vi "Configure Control AO Split.vi"(0 "VISA resource name":refnum<visa-resource-name>, 1 "Output 0% value of Line Point":dbl min=-1000.0 max=2000.0 step=1.0 format="%.1f", 5 "Unit No. (0)":i32 min=0 max=6, 7 "Module No.(0)":i32 min=0 max=9, 9 "AO No.(1)":i32=1 min=1 max=2, 11 "error in (no error)":errorcluster, 12 "Line Mode(false)":bool, 13 "Output 100% value of Line Point":dbl=100.0 min=-1000.0 max=2000.0 format="%.1f") -> (4 "VISA resource name out":refnum<visa-resource-name>, 6 "AO No.":i32, 8 "Unit No.":i32, 10 "Module No.":i32, 15 "error out":errorcluster)   [LabVIEW 2020, in "Yokogawa GX Series.lvlib"]
doc: "Set AO Split of the PID Module.\n\nCommand: SCtrlSplitAO"
uses:
  <instrlib>/Yokogawa GX Series/Yokogawa GX Series.lvlib
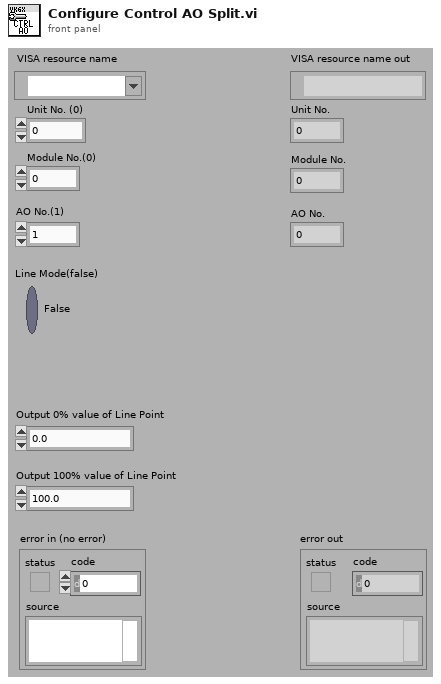
[diagram p1: front panel]
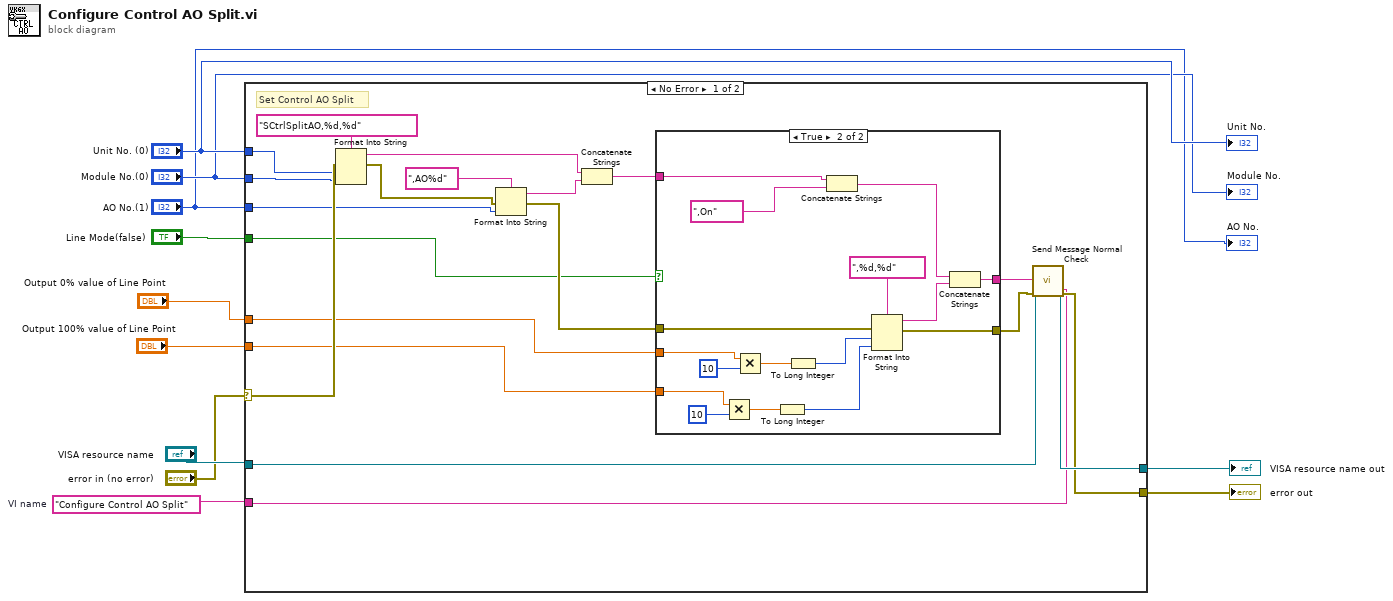
[diagram p0: block diagram]
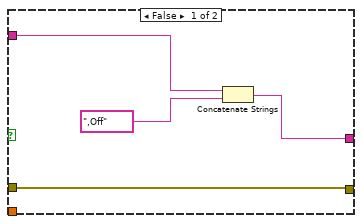
[diagram p2: hidden frame]
diagram:
  w7 = "Configure Control AO Split"  # VI name
  n1 = case shown="No Error" "error in (no error)" {
    selector: "error in (no error)" -> [w27 w52]
    tunnel: [w31 w53] -> w11
    tunnel: [w30 w52] -> w10
    tunnel: "VISA resource name" -> [w29 w53]
    tunnel: w7 -> [w26 _]
    tunnel: "Unit No. (0)" -> [w25 _]
    tunnel: "Module No.(0)" -> [w24 _]
    tunnel: "AO No.(1)" -> [w22 _]
    tunnel: "Output 0% value of Line Point" -> [w15 _]
    tunnel: "Line Mode(false)" -> [w12 _]
    tunnel: "Output 100% value of Line Point" -> [w14 _]
    frame No Error {
      # "Set Control AO Split"
      n2 = Format Into String(format string="SCtrlSplitAO,%d,%d", error in=w27, w25, w24) -> (resulting string=w20:string, error out=w21:errorcluster)  [unwired: 1 in]
      n3 = Format Into String(format string=",AO%d", error in=w21, w22) -> (resulting string=w19:string, error out=w17:errorcluster)  [unwired: 1 in]
      n4 = Concatenate Strings(w20, w19) -> (w18:string)
      n5 = case shown="True" w12 {
        tunnel: w18 -> [w32 w49]
        tunnel: w17 -> [w34 w48]
        tunnel: [w34 w47] -> w16
        tunnel: w15 -> [_ w39]
        tunnel: w14 -> [_ w38]
        tunnel: [w33 w37] -> w13
        frame False {
          n6 = Concatenate Strings(w32, ",Off") -> (w33:string)
        }
        frame True {
          n7 = Multiply(x=w38, y=10) -> (x*y=w41:dbl)
          n8 = Multiply(x=w39, y=10) -> (x*y=w44:dbl)
          n9 = To Long Integer(number=w41) -> (32bit integer=w40:i32)
          n10 = To Long Integer(number=w44) -> (32bit integer=w43:i32)
          n11 = Concatenate Strings(w49, ",On") -> (w46:string)
          n12 = Format Into String(format string=",%d,%d", error in=w48, w43, w40) -> (resulting string=w50:string, error out=w47:errorcluster)  [unwired: 1 in]
          n13 = Concatenate Strings(w46, w50) -> (w37:string)
        }
      }
      n14 = call <instrlib>:"Send Message Normal Check.vi"("Source (\"\")"=w26, "error in (no error)"=w16, "Send Message (\"\")"=w13, "VISA resource name"=w29) -> ("error out"=w30:errorcluster, "VISA resource name out"=w31:refnum<visa-resource-name>)  [unwired: 2 in, 4 out]
    }
    frame Error {
    }
  }
  "error out" <- w10
  "VISA resource name out" <- w11
  "Unit No." <- "Unit No. (0)"
  "Module No." <- "Module No.(0)"
  "AO No." <- "AO No.(1)"
